vi "LocalAppData Get or Create App Directory.vi"(8 "error in (no error)":errorcluster, 11 "Relative Path":path) -> (0 "error out":errorcluster, 3 "Output File Path":path)   [LabVIEW 2020, in "RxnRover.lvlib" / "File IO.lvlib" / "LocalAppData Utilities.lvlib"]
doc: "Create or access a local app directory given a relative path(String) EX: appname/appdirectory\n\nLocates the correct system-specfic base directory for state data %LOCALAPPDATA(WIndows) or $XDG_STATE_HOME(Linux) or ~/Library/Application Support(Mac OS) and appends the relative path\nCreates the directory if it does not exist. \nCompliant with XKG Base Directory Specification \n\nCreated 5/20/2025 - Labview 2020\nRxnRover"
uses:
  LocalAppData Utilities.lvlib
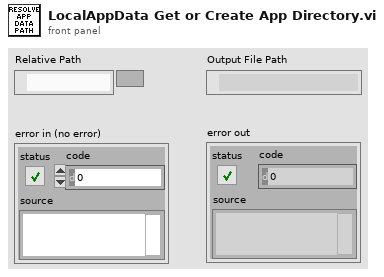
[diagram p1: front panel]
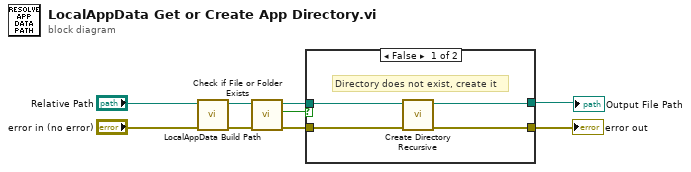
[diagram p0: block diagram]
diagram:
  n1 = call "LocalAppData Build Path.vi"("error in (no error)"="error in (no error)", "Relative path"="Relative Path") -> ("error out"=w5:errorcluster, "Full Path"=w9:path)  [unwired: 8 in]
  n2 = call <vilib>:"Check if File or Folder Exists.vi"("error in (no error)"=w5, "path"=w9) -> ("error out"=w6:errorcluster, "file or folder exists?"=w8:bool, "dup path"=w7:path)  [unwired: 7 in]
  n3 = case shown="False" w8 {
    tunnel: w7 -> [w13 w15]
    tunnel: [w12 w15] -> w2
    tunnel: w6 -> [w11 w14]
    tunnel: [w10 w14] -> w3
    frame False {
      # "Directory does not exist, create it"
      n4 = call <vilib>:"Create Directory Recursive.vi"("error in (no error)"=w11, "directory"=w13) -> ("error out"=w10:errorcluster, "directory copy"=w12:path)  [unwired: 3 in, 1 out]
    }
    frame True {
      # "Directory already exists pass the full path"
    }
  }
  "error out" <- w3
  "Output File Path" <- w2
